vi "TEMP_CONTROL.vi"() -> ()   [LabVIEW 2023]
uses:
  <vilib>/MakerHub/LINX/Public/Sensors/Temperature/TCN75A/Resolution.ctl
  <vilib>/MakerHub/LINX/Public/Peripherals/Digital/Digital Write 1 Chan.vi
  <vilib>/MakerHub/LINX/Public/Peripherals/PWM/PWM Set Duty Cycle 1 Chan.vi
  <vilib>/MakerHub/LINX/Public/Peripherals/Digital/Digital Write N Chans.vi
  <vilib>/MakerHub/LINX/Private/Local IO/LinxDigitalWrite.vi
  <vilib>/MakerHub/LINX/Public/Utilities/Check Channel.vi
  <vilib>/MakerHub/LINX/Public/Utilities/Open Serial.vi
  <vilib>/MakerHub/LINX/Private/Utilties/Generate Error.vi
  <vilib>/MakerHub/LINX/Public/Peripherals/PWM/PWM Set Duty Cycle N Chans.vi
  <vilib>/MakerHub/LINX/LMH-LINX.lvlib
  <vilib>/MakerHub/LINX/Public/Sensors/Temperature/TCN75A/TCN75A.lvlib
panel:
  out "Measure and control":bool
  out "String":string
  in  "Tab Control":enum32{"Page 1"}(tab)
  out "Pont H":bool
  out "Situation":string
  out "?":dbl(graph)
  out "?":dbl(slide) scale=-30.0..90.0
  out "Temp C":dbl
  out "Chauffe":bool
  in  "Consigne":dbl
  out "Refroidir":bool
  in  "?":bool
  in  "Serial Port":refnum<visa-resource-name>="N/A"
  in  "Resolution":T1
  # "Mise en place d'un banc de calibration d'une caméra thermique"
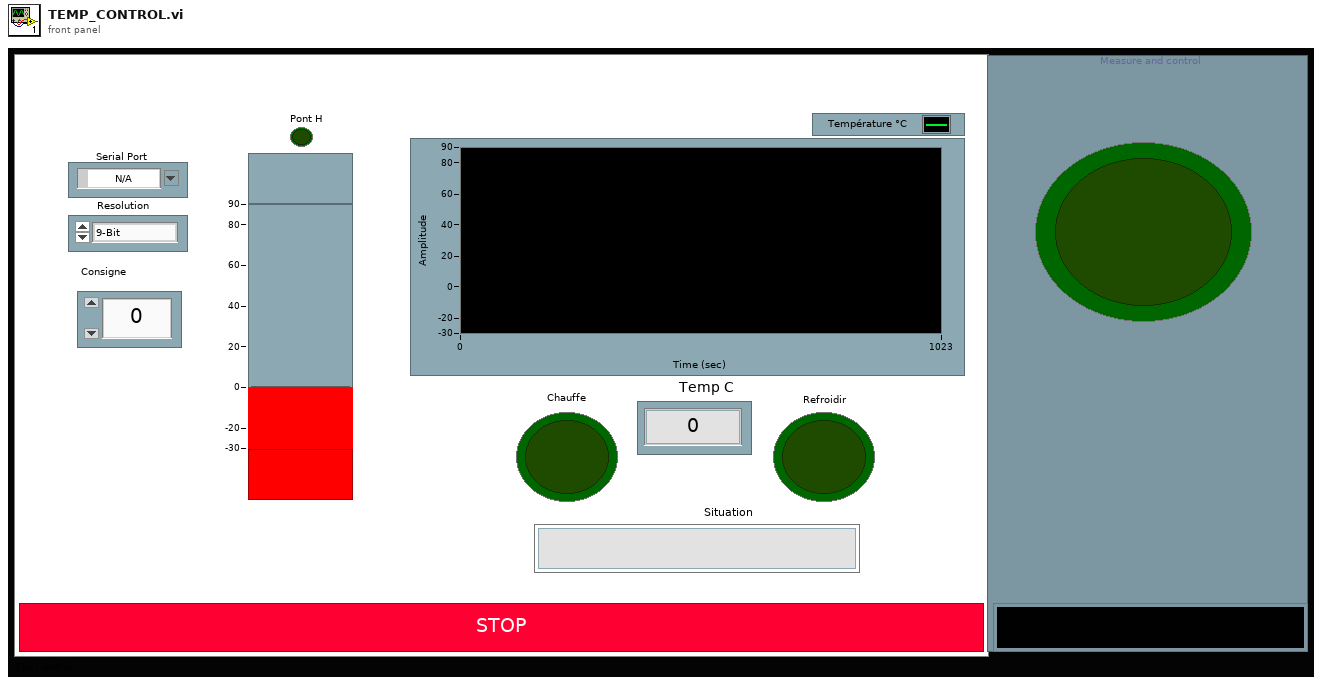
[diagram p1: front panel]
types:
  T1 = typedef "LMH-LINX.lvlib/TCN75A.lvlib/Resolution.ctl" = enum8{"9-Bit", "10-Bit", "11-Bit", "12-Bit"}
  T2 = typedef "LMH-LINX.lvlib/LINX Ref.ctl" = cluster{"IO":T3, "Interface":T4, "LINX Device Config":T5}
  T3 = typedef "LMH-LINX.lvlib/Platform.ctl" = enum16{"Remote", "Local"}
  T4 = typedef "LMH-LINX.lvlib/Interface.ctl" = enum16{"Serial", "TCP"}
  T5 = typedef "LMH-LINX.lvlib/Device.lvlib/LINX Device Config.ctl" = cluster{"Interface":T4, "COM Port":refnum<visa-resource-name>, "TCP Configuration":T6, "Device Family":u8, "Device ID":u8, "Device Name":string, "TCP Ref":refnum<k5>, "Channels":T7}
  T6 = typedef "LMH-LINX.lvlib/Device.lvlib/TCP Config.ctl" = cluster{"IP Address":string, "Port":u16}
  T7 = typedef "LMH-LINX.lvlib/Channels.ctl" = cluster{"DI":u8[], "DO":u8[], "AI":u8[], "AO":u8[], "PWM":u8[], "QE":u8[], "UART":u8[], "I2C 2":u8[], "SPI":u8[], "CAN":u8[], "Servo":u8[], "AI Ref (V)":dbl, "AI Resolution (Bits)":u8, "AO Ref (V)":dbl, "AO Resolution (Bits)":u8}
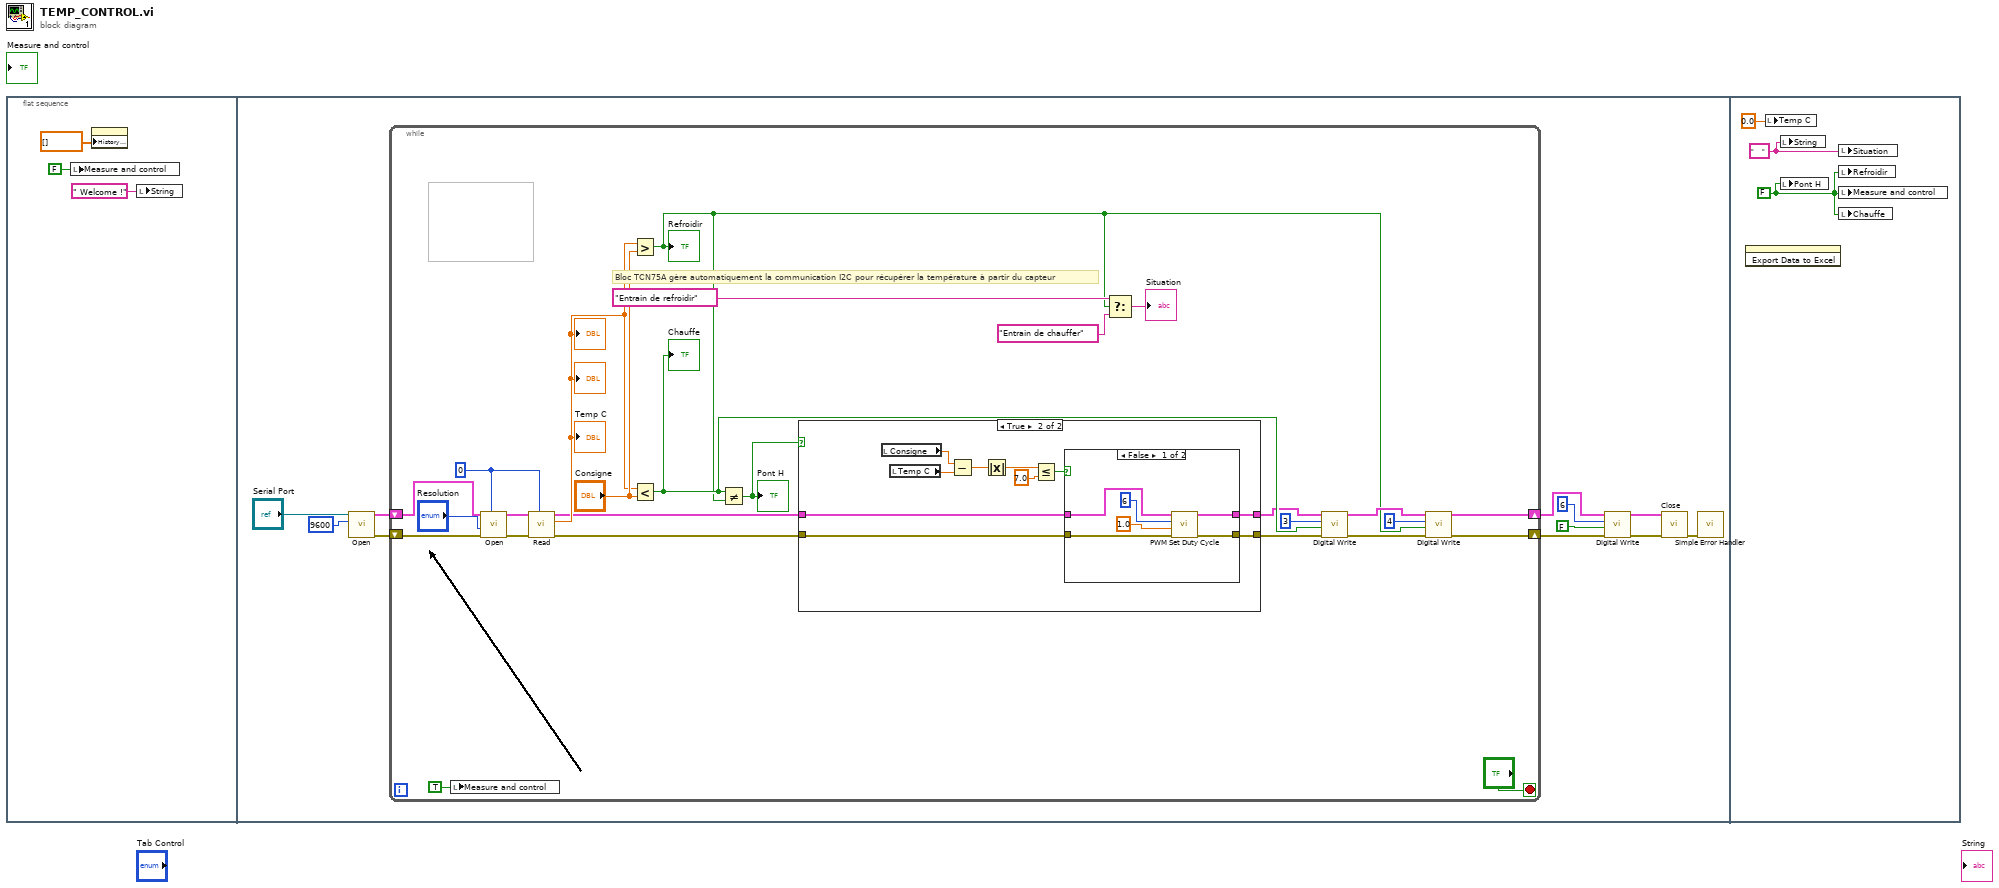
[diagram p0: block diagram]
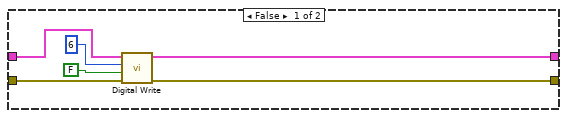
[diagram p2: hidden frame]
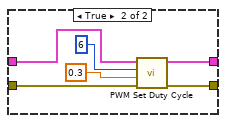
[diagram p3: hidden frame]
diagram:
  n1 = flat-sequence {
    frame #0 {
      n2 = local write "Measure and control"(FALSE ("LED")) -> ()
      n3 = property class="WFChart (strict)"("History Data"=dbl[] []) -> ()  [unwired: 2 in, 2 out]
      n4 = local write "String"(" Welcome !" ("String")) -> ()
    }
    frame #1 {
      n5 = call-poly <vilib>:"Open.vi"("Baud Rate Override"=u32 9600, "Serial Port"="Serial Port") -> ("Error Out"=w13:errorcluster, "LINX Resource"=w14:T2)  [unwired: 7 in, 1 out]
      n6 = while {
        shift-right: [w36] -> w9
        shift-left: w14 -> [w30]
        shift-right: [w35] -> w6
        shift-left: w13 -> [w29]
        stop <- "?" stop-if-true
        w31 = u8 0 ("I2C Channel (0)")
        # "Bloc TCN75A gère automatiquement la communication I2C pour récupérer la température à partir du capteur"
        n7 = local write "Measure and control"(TRUE ("LED")) -> ()
        n8 = call <vilib>:"Open.vi"("I2C Channel (0)"=w31, "Error In"=w29, "Resolution"="Resolution", "LINX Resource"=w30) -> ("Error Out"=w33:errorcluster, "LINX Resource"=w32:T2)  [unwired: 6 in]
        n9 = call <vilib>:"Read.vi"("I2C Channel (0)"=w31, "Error In"=w33, "LINX Resource"=w32) -> ("Error Out"=w17:errorcluster, "Temp C"=w23:dbl, "LINX Resource"=w18:T2)  [unwired: 5 in, 1 out]
        "?" <- w23
        "?" <- w23
        "Temp C" <- w23
        n10 = Greater?(x=w23, y="Consigne") -> (0:w21:bool)
        "Refroidir" <- w21
        n11 = Less?(x=w23, y="Consigne") -> (x < y?=w22:bool)
        "Chauffe" <- w22
        n12 = Not Equal?(x=w22, y=w21) -> (x != y?=w19:bool)
        "Pont H" <- w19
        n13 = case shown="True" w19 {
          tunnel: w18 -> [w46 w55]
          tunnel: w17 -> [w45 w56]
          tunnel: [w44 w53] -> w16
          tunnel: [w43 w54] -> w15
          frame False {
            n14 = call-poly <vilib>:"Digital Write.vi"("Error In"=w45, "Output Value"=FALSE, "DO Channel"=u8 6, "LINX Resource"=w46) -> ("Error Out"=w43:errorcluster, "LINX Resource"=w44:T2)  [unwired: 6 in]
          }
          frame True {
            n15 = local read "Consigne"() -> (w52:dbl)
            n16 = local read "Temp C"() -> (w51:dbl)
            n17 = Subtract(x=w52, y=w51) -> (x-y=w50:dbl)
            n18 = Absolute Value(x=w50) -> (abs(x)=w49:dbl)
            n19 = Less Or Equal?(x=w49, y=7.0) -> (x <= y?=w47:bool)
            n20 = case shown="False" w47 {
              tunnel: w56 -> [w61 w68]
              tunnel: w55 -> [w62 w66]
              tunnel: [w60 w65] -> w54
              tunnel: [w59 w64] -> w53
              frame False {
                n21 = call-poly <vilib>:"PWM Set Duty Cycle.vi"("Error In"=w61, "Duty Cycle (0-1)"=1.0, "PWM Channel"=u8 6, "LINX Resource"=w62) -> ("Error Out"=w60:errorcluster, "LINX Resource"=w59:T2)  [unwired: 6 in]
              }
              frame True {
                n22 = call-poly <vilib>:"PWM Set Duty Cycle.vi"("Error In"=w68, "Duty Cycle (0-1)"=0.3, "PWM Channel"=u8 6 ("DI Channel"), "LINX Resource"=w66) -> ("Error Out"=w65:errorcluster, "LINX Resource"=w64:T2)  [unwired: 6 in]
              }
            }
          }
        }
        n23 = Select(t="Entrain de refroidir", s=w21, f="Entrain de chauffer") -> (s? t:f=→"Situation":string)
        n24 = call-poly <vilib>:"Digital Write.vi"("Error In"=w15, "Output Value"=w22, "DO Channel"=u8 3, "LINX Resource"=w16) -> ("Error Out"=w39:errorcluster, "LINX Resource"=w40:T2)  [unwired: 6 in]
        n25 = call-poly <vilib>:"Digital Write.vi"("Error In"=w39, "Output Value"=w21, "DO Channel"=u8 4, "LINX Resource"=w40) -> ("Error Out"=w35:errorcluster, "LINX Resource"=w36:T2)  [unwired: 6 in]
      }
      n26 = call-poly <vilib>:"Digital Write.vi"("Error In"=w6, "Output Value"=FALSE, "DO Channel"=u8 6, "LINX Resource"=w9) -> ("Error Out"=w7:errorcluster, "LINX Resource"=w8:T2)  [unwired: 6 in]
      n27 = call <vilib>:"Close.vi"("Error In"=w7, "LINX Resource"=w8) -> ("Error Out"=w11:errorcluster)  [unwired: 9 in]
      n28 = call <vilib>:"Simple Error Handler.vi"("error in (no error)"=w11) -> ()  [unwired: 4 in, 5 out]
    }
    frame #2 {
      w69 = FALSE ("Pont H")
      w71 = "    " ("String")
      n29 = invoke class="WFChart (strict)" method="Export Data to Excel"() -> ()  [unwired: 3 in, 3 out]
      n30 = local write "Temp C"(0.0 ("Temp C")) -> ()
      n31 = local write "String"(w71) -> ()
      n32 = local write "Pont H"(w69) -> ()
      n33 = local write "Situation"(w71) -> ()
      n34 = local write "Refroidir"(w69) -> ()
      n35 = local write "Measure and control"(w69) -> ()
      n36 = local write "Chauffe"(w69) -> ()
    }
  }
